vi "SUB_VI_scrittura_messaggio_array.vi"(8 "Errore in ingresso":errorcluster, 10 "Segnale da inviare":waveform(dbl), 11 "TCP Network Connection in":refnum<k5>) -> (0 "Errore uscita":errorcluster, 3 "TCP Network Connection out":refnum<k5>)   [LabVIEW 2023]
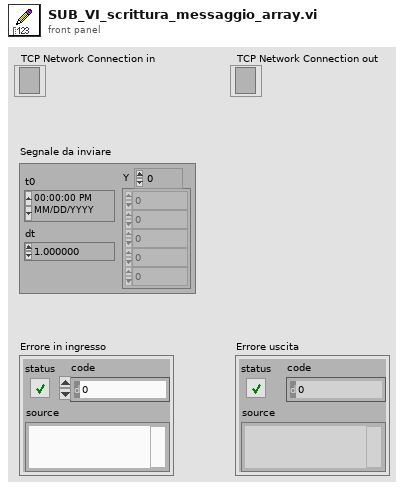
[diagram p1: front panel]
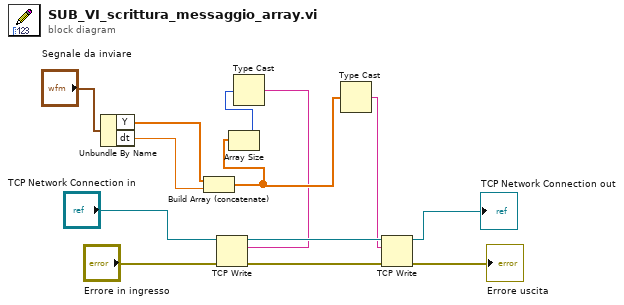
[diagram p0: block diagram]
diagram:
  n1 = Unbundle By Name("Segnale da inviare") -> ("Y"=w10:dbl[], "dt"=w1:dbl)
  n2 = Build Array (concatenate)(w10, w1) -> (w9:dbl[])
  n3 = Array Size(array=w9) -> (size(s)=w6:i32)
  n4 = Type Cast(x=w6) -> (*(type *) &x=w2:string)  [unwired: 1 in]
  n5 = TCP Write(connection ID="TCP Network Connection in", data in=w2, error in (no error)="Errore in ingresso") -> (connection ID out=w4:refnum<k5>, error out=w5:errorcluster)  [unwired: 1 in, 1 out]
  n6 = Type Cast(x=w9) -> (*(type *) &x=w3:string)  [unwired: 1 in]
  n7 = TCP Write(connection ID=w4, data in=w3, error in (no error)=w5) -> (connection ID out=→"TCP Network Connection out":refnum<k5>, error out=→"Errore uscita":errorcluster)  [unwired: 1 in, 1 out]
